vi "Drivetrain Loop.vi"(6 "Reset the clock":bool, 8 "In 4":dbl, 9 "In 3":dbl, 10 "In 2":dbl, 11 "In 1":dbl) -> (0 "Out 4":dbl, 1 "Out 3":dbl, 2 "Out 2":dbl, 3 "Out 1":dbl)   [LabVIEW 2015]
uses:
  Common Code/Drivetrain Modes.ctl
  Common Code/Change Detect Boolean.vi
  Robot Global Data.vi
  <vilib>/Rock Robotics/WPI/Solenoid/Deprecated/WPI_SolenoidSetBool.vi
panel:
  out "Modes":T1=enum."Goal Vision Targeting"
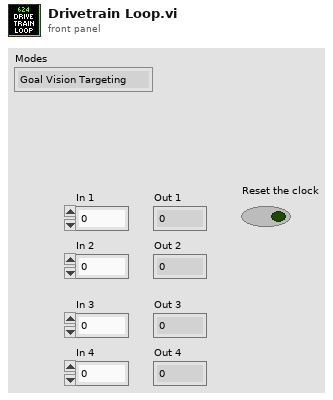
[diagram p1: front panel]
types:
  T1 = typedef "Drivetrain Modes.ctl" = enum16{"Tank", "Climb", "Manual", "Goal Vision Targeting", "PID Distance Drive", "Hybrid", "Gyro Steer"}
  T2 = typedef "Drivetrain Commands.ctl" = cluster{"Y Power":dbl, "Turn Power":dbl, "2nd Gear?":bool, "Modes":T1, "Heading Target":dbl, "X Max Speed":dbl, "Y Max Speed":dbl, "X Min Speed":dbl, "Y Min Speed":dbl, "Y Target":dbl, "Max Accel":dbl, "Max Velocity":dbl, "Y Power 2":dbl, "Pivot Speed":dbl}
  T3 = typedef "WPI_DriverStationRobotMode2.ctl" = enum16{"Autonomous Disabled", "Autonomous Enabled", "Teleop Disabled", "Teleop Enabled", "Disconnected", "Finish", "Test Disabled", "Test Enabled", "Emergency Stopped"}
  T4 = typedef "Goal Vision Packet.ctl" = cluster{"Distance":dbl, "Center X":dbl, "Center Y":dbl, "Found Target?":bool, "Robot Center":dbl, "Angle":dbl}
  T5 = typedef "Dashboard Control Data.ctl" = cluster{"Shooter Presets":T6, "Encoder Control":T8, "Steer PID output":cluster{"output high":dbl, "output low":dbl}, " Steer PID gains":cluster{"proportional gain (Kc)":dbl, "integral time (Ti, min)":dbl, "derivative time (Td, min)":dbl}, "Drivetrain Settings":T9, "Vision Packet":T4, "Dashboard Drivetrain Command":T10, "Info/Command Cluster":T12, "Ball Vision Packet":T13, "Intake Presets":T15, "Intake Encoder Control":T17, "Climb Presets":T18, "Goal Output Range":cluster{"output high":dbl, "output low":dbl}, "Enabled Systems":T19, "Auton Presets":T20, "Pressure M":dbl, "Pressure B":dbl, "Vision Timeout":dbl, "Auto-Shift":T21}
  T6 = typedef "Shooter Presets.ctl" = cluster{"Batter Shot":T7, "Deep Middle":T7, "Manual Shot":T7, "Left Ticks Per Rotation":dbl, "Right Ticks Per Rotation":dbl, "Low Bar Shot":T7, "Shooter RPM Tolerance":dbl, "Trigger Power":dbl, "Fire from Load Delay":i32, "Max Angle":dbl, "Min Angle":dbl, "Angle PID gains":cluster{"P":dbl, "I":dbl, "D":dbl}, "Angle Output":cluster{"output high":dbl, "output low":dbl}, "Shooter Angle Tolerance":dbl, "Vision Shoot x^2":dbl, "Vision Shoot x":dbl, "Feed Forward Max Accel":dbl, "Feed Forward Kv":dbl, "Backwards Trigger":dbl, "Shot Finish Delay (ms)":dbl, "Angle Max Current":dbl, "Angle Current Trip Time":dbl, "Intake Angle":dbl, "Vision Shoot c":dbl, "Reset?":bool, "Button Release Delay":dbl, "Angle Pot x":dbl, "Angle Pot c":dbl, "Ignore Angle?":bool, "Max RPM":dbl, "Safty Frist Angle":dbl, "Intake Danger Height":dbl, "Angle Pot B":i32, "Angle Pot M":dbl, "FF Finish RPM":dbl, "RPM PID Right":cluster{"P":dbl, "I":dbl, "D":dbl, "FF":dbl}, "RPM PID Left":cluster{"P":dbl, "I":dbl, "D":dbl, "FF":dbl}, "Backwards RPM":dbl, "Vision RPM":dbl, "Run Wheels Backward Delay":u32, "Cleat Shot":T7, "Vision Far RPM":dbl, "Vision Far Distance":dbl, "Vision Far Angle":dbl}
  T7 = typedef "Shot Presets.ctl" = cluster{"L":dbl, "R":dbl, "A":dbl}
  T8 = typedef "Encoder Control.ctl" = cluster{"Right Tick Constant":dbl, "Left Tick Constant":dbl, "Reset?":bool, "Y Dist":cluster{"PID gains":cluster{"proportional gain (Kc)":dbl, "integral time (Ti, min)":dbl, "derivative time (Td, min)":dbl}}, "Y Stop Thresh":dbl, "Y Stop Speed":dbl}
  T9 = typedef "Drivetrain Settings.ctl" = cluster{"Gyro Tolerance":dbl, "Throttle Ramp (ms)":dbl, "Kv":dbl, "Ka":dbl, "Feed Forward P":dbl, "Feed Forward D":dbl, "Goal Vision PID gains":cluster{"proportional gain (Kc)":dbl, "integral time (Ti, min)":dbl, "derivative time (Td, min)":dbl}, "Goal Detection Window":dbl, "Creep Rate":dbl, "Vision Throttle Threshold":dbl, "Min Turn Output":dbl, "Left Batter Angle":dbl, "Right Batter Angle":dbl}
  T10 = typedef "Dashboard Drivetrain Command.ctl" = cluster{"Drivetrain Vision":T11}
  T11 = typedef "Drivetrain Vision.ctl" = cluster{"Goal Window":dbl, "Ball Window":dbl}
  T12 = typedef "Ball Tracking Command Cluster.ctl" = cluster{"Distance to Ball":dbl, "Desired Angle":dbl, "Command":enum16{"Turn to Ball", "Turn to Angle", "Get Distance"}, "Pixels from Center":dbl}
  T13 = typedef "Ball Vision Packet.ctl" = cluster{"Ball Detected?":bool, "Distance to Ball":dbl, "Desired Angle":dbl, "Pixels from Center":dbl, "Tracking mode":T14}
  T14 = typedef "Tracking Mode.ctl" = enum16{"Turn to Ball", "Turn to Angle"}
  T15 = typedef "Intake Presets.ctl" = cluster{"Intake Speed":dbl, "Outake Speed":dbl, "Low Height":dbl, "Half Height":dbl, "High Idle Height":dbl, "Angle Speed":dbl, "Angle Tolerance":dbl, "Encoder Scale":dbl, "Load Height":dbl, "Output Range":T16, "Rotation Power Max/Min":dbl, "MaxCurrent":dbl, "Intake Trip Time":dbl, "Idle Height":dbl, "Max Height":dbl, "Reset Encoders?":bool, "PID gains":cluster{"proportional gain (Kc)":dbl, "integral time (Ti, min)":dbl, "derivative time (Td, min)":dbl}, "Intake Stop Delay":u32, "Settle Time":dbl, "Settle Wait Time":dbl, "Pull Up Delay":dbl}
  T16 = typedef "Drivetrain Output Range.ctl" = cluster{"output high":dbl, "output low":dbl}
  T17 = typedef "IntakeEcoderControl.ctl" = cluster{"Arm Tick Constant":dbl, "Reset?":bool, "Y Dist":cluster{"PID gains":cluster{"proportional gain (Kc)":dbl, "integral time (Ti, min)":dbl, "derivative time (Td, min)":dbl}}, "Y Stop Thresh":dbl, "Y Stop Speed":dbl}
  T18 = typedef "Climb Presets.ctl" = cluster{"Pull Power":dbl, "Extend Power":dbl}
  T19 = typedef "Enabled Systems.ctl" = cluster{"Shoot":bool, "Intake":bool, "DT":bool, "Gyro":bool, "100ms":bool, "US":bool}
  T20 = typedef "Autonomous Presets.ctl" = cluster{"Pitch Limit":dbl, "Roll Limit":dbl, "Start Position":dbl, "Cross Position":dbl}
  T21 = typedef "Auto Shift Cluster.ctl" = cluster{"Delay":dbl, "Speed Thresh":dbl, "Upshift Accel":dbl, "Upshift Throttle":dbl, "Upshift Throttle Accel":dbl, "Downshift Throttle":dbl, "Downshift Throttle Accel":dbl, "Pressure Threshold":dbl}
  T22 = typedef "Dist Drive Status.ctl" = cluster{"Y In Range":bool, "X In Range":bool, "Gyro In Range":bool, "Y Dist":dbl, "X Dist":dbl, "Gyro":dbl}
  T23 = typedef "WPI_MotorControlDeviceRef.ctl" = cluster{"DeviceStatus":errorcluster, "Type":T24, "PWM":cluster{"PWM Channel":T25, "DeadBand":T26}, "CAN":cluster{"Device Number":u8, "Control Mode":T27, "Semaphore":T28, "Max Vout":dbl, "TalonSRX Control Mode":T29}, "Invert":bool}
  T24 = typedef "WPI_MotorControlType.ctl" = enum16{"PWM", "CAN", "CANTalonSRX"}
  T25 = typedef "FPGA_DIOPWMChannel.ctl" = enum8{"PWM 0", "PWM 1", "PWM 2", "PWM 3", "PWM 4", "PWM 5", "PWM 6", "PWM 7", "PWM 8", "PWM 9", "PWM MXP 0", "PWM MXP 1", "PWM MXP 2", "PWM MXP 3", "PWM MXP 4", "PWM MXP 5", "PWM MXP 6", "PWM MXP 7", "PWM MXP 8", "PWM MXP 9", "Invalid"}
  T26 = typedef "WPI_PWMDeadband.ctl" = cluster{"Name":string, "maxPositivePwm":i32, "minPositivePwm":i32, "centerPwm":i32, "maxNegativePwm":i32, "minNegativePwm":i32, "angularRange":u16}
  T27 = typedef "WPI_CANJaguar_ControlMode.ctl" = enum8{"Percent VBus", "Current", "Speed", "Position", "Voltage"}
  T28 = typedef "Semaphore RefNum" = refnum<k1>
  T29 = typedef "WPI_CANTalonSRX_APIControlMode.ctl" = enum8{"Percent VBus", "Speed", "Position", "Slave", "Unchanged / Invalid", "Voltage Compensation", "Current", "Motion Profile"}
  T30 = typedef "WPI_SolenoidDevRef.ctl" = cluster{"DevStatus":errorcluster, "Pneumatics Control Module":u8, "Forward Solenoid Channel":T31, "Reverse Solenoid Channel":T31}
  T31 = typedef "WPI_SolenoidChannel.ctl" = enum8{"Solenoid 0", "Solenoid 1", "Solenoid 2", "Solenoid 3", "Solenoid 4", "Solenoid 5", "Solenoid 6", "Solenoid 7", "Invalid"}
  T32 = typedef "Drivetrain Status Cluster.ctl" = cluster{"Modes":T1, "Y (Throttle)":dbl, "X (Steer)":dbl, "Gyro In Range?":bool, "Distance Drive Finished?":bool, "Stop Eject Lockout":bool, "Dist Drive Status":T22, "Y Target":dbl, "Heading Target":dbl, "Vision Target Aligned?":bool, "Gear":dbl, "1st Gear Time":dbl, "2nd Gear Time":dbl, "1st Gear Shifts":dbl, "2nd Gear Shifts":dbl}
  T33 = typedef "Climb Status Cluster.ctl" = cluster{"Pull Power":dbl, "Unpin Power":dbl, "PTO Engaged?":bool, "Climb Mode":T34}
  T34 = typedef "Climb Mode.ctl" = enum16{"Auto", "Semi-Auto", "Manual"}
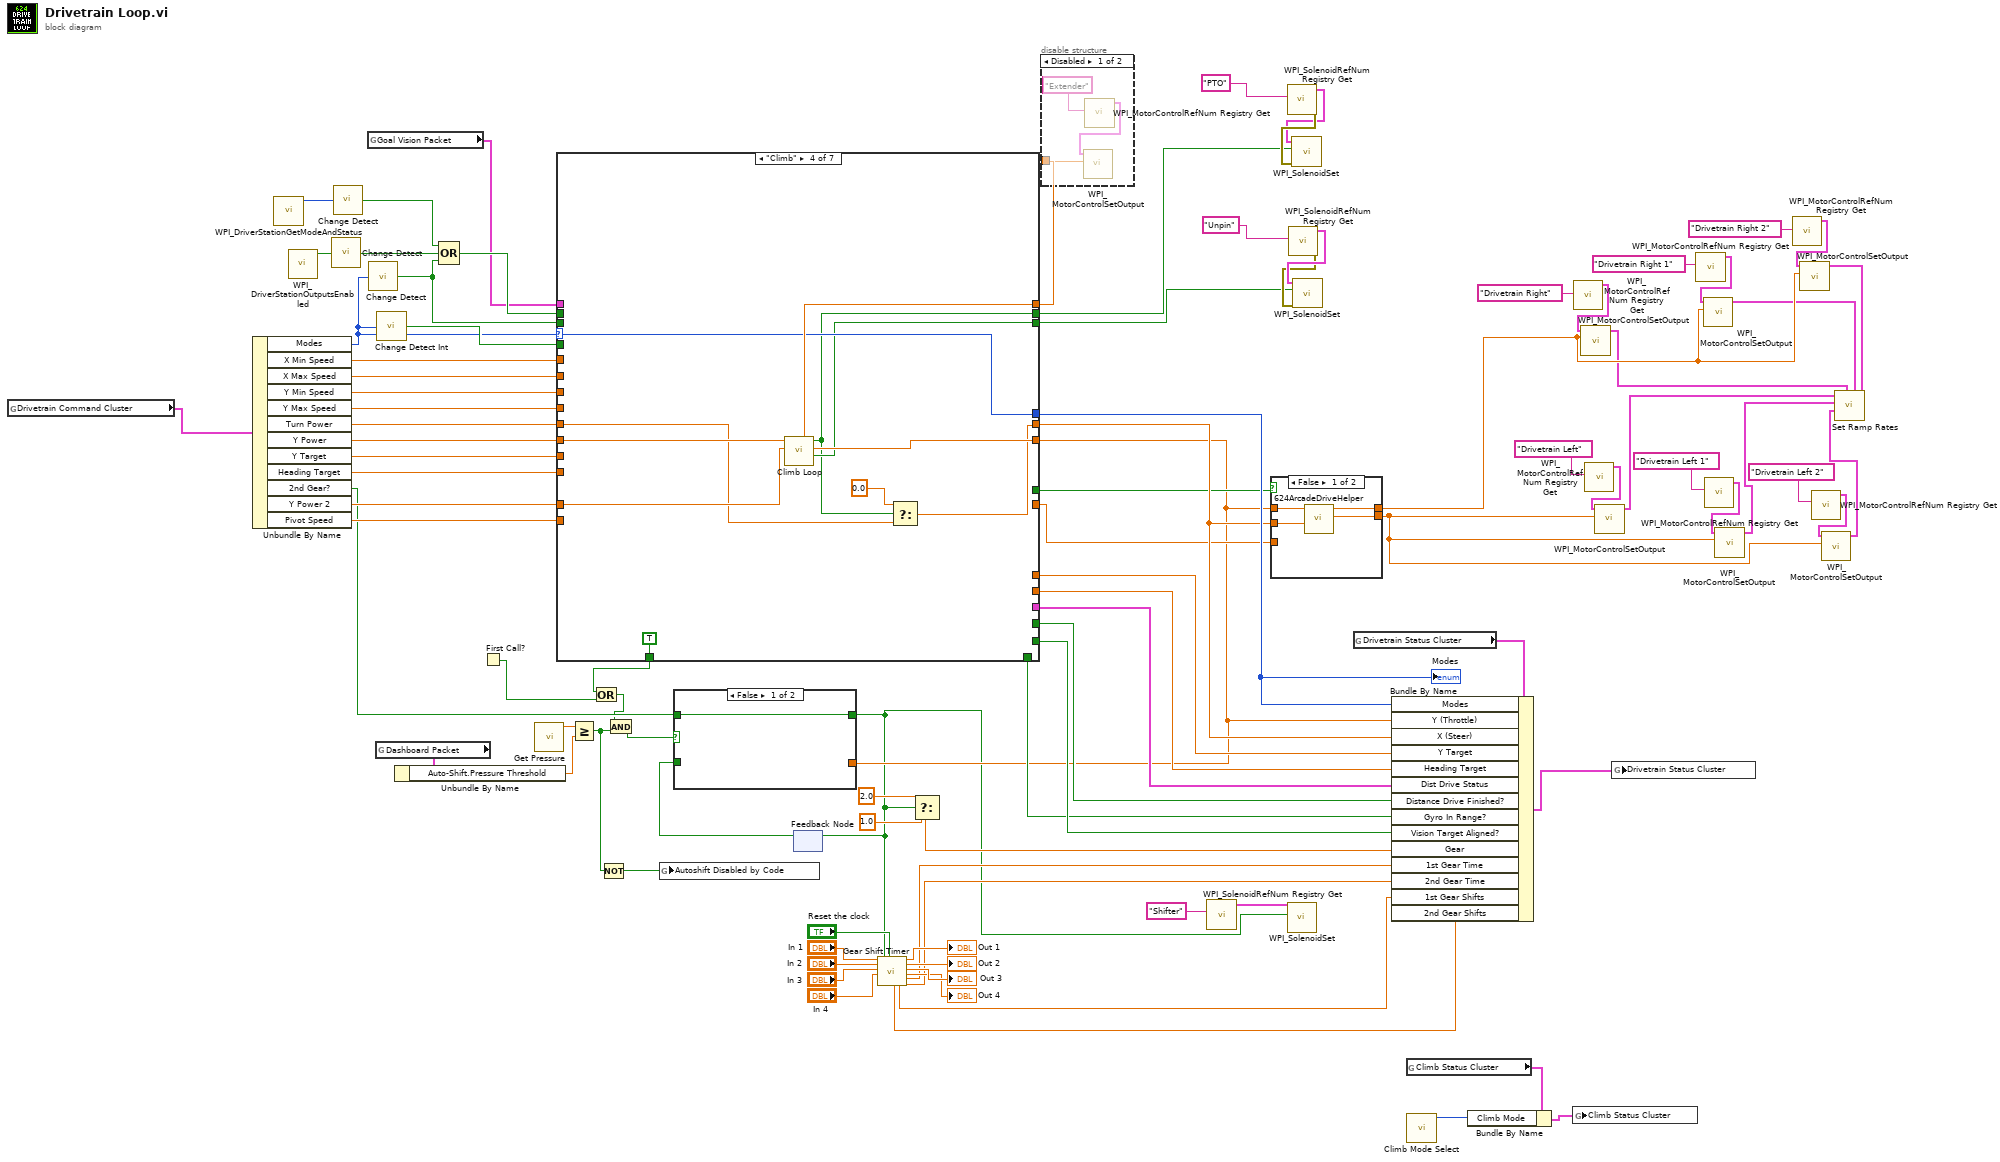
[diagram p0: block diagram]
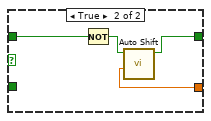
[diagram p2: hidden frame]
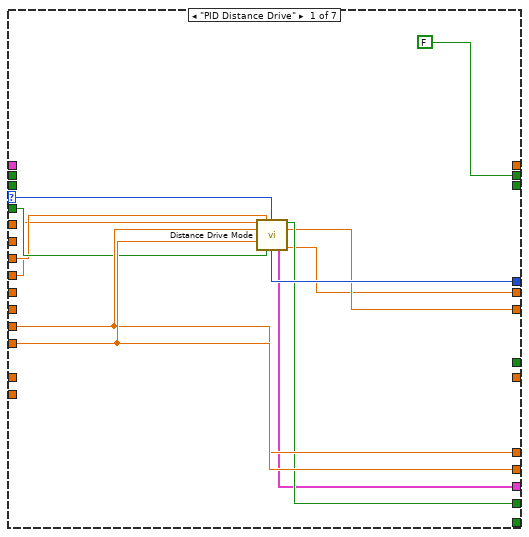
[diagram p4: hidden frame]
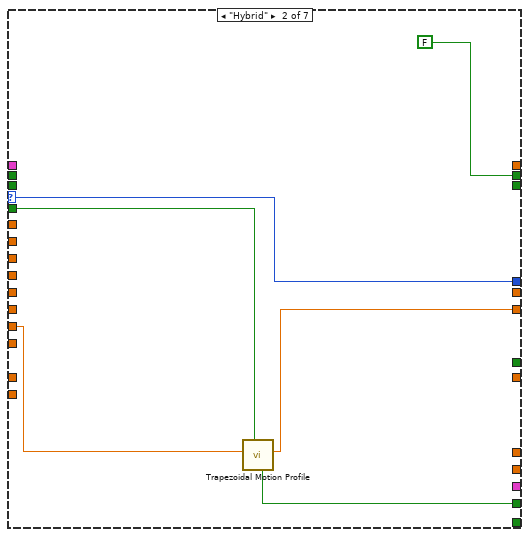
[diagram p5: hidden frame]
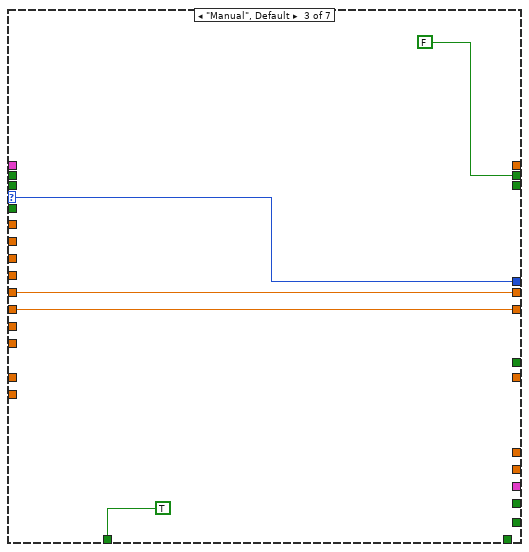
[diagram p6: hidden frame]
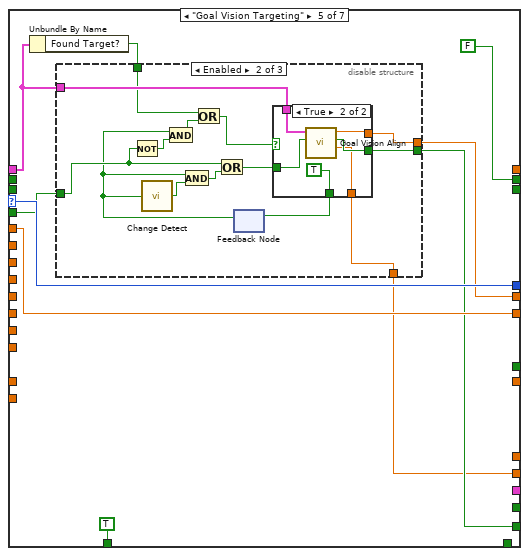
[diagram p7: hidden frame]
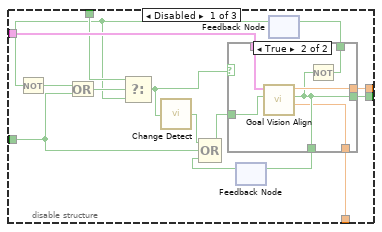
[diagram p8: hidden frame]
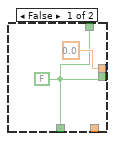
[diagram p9: hidden frame]
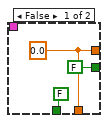
[diagram p10: hidden frame]
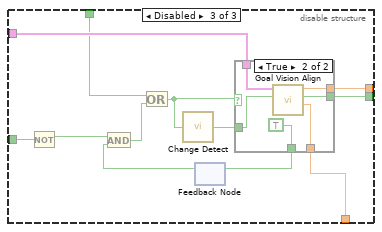
[diagram p11: hidden frame]
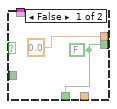
[diagram p12: hidden frame]
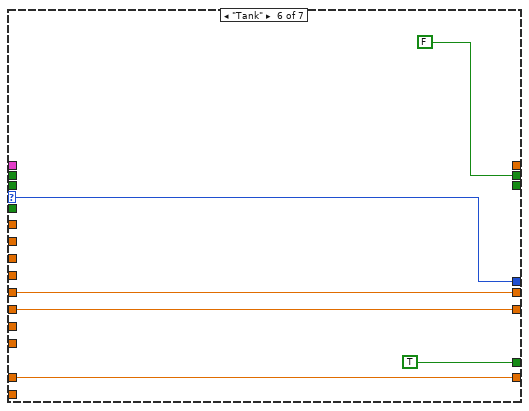
[diagram p13: hidden frame]
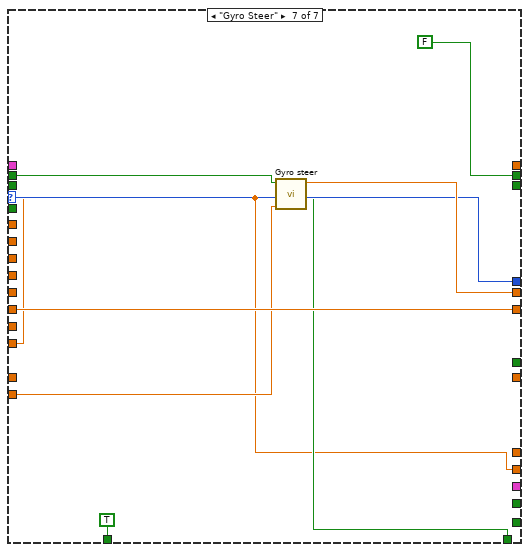
[diagram p14: hidden frame]
diagram:
  n1 = global read "Robot Global Data.vi" "Drivetrain Command Cluster"() -> (w60:T2)
  n2 = Unbundle By Name(w60) -> ("Modes"=w45:T1, "X Min Speed"=w69:dbl, "X Max Speed"=w68:dbl, "Y Min Speed"=w67:dbl, "Y Max Speed"=w66:dbl, "Turn Power"=w65:dbl, "Y Power"=w64:dbl, "Y Target"=w63:dbl, "Heading Target"=w62:dbl, "2nd Gear?"=w13:bool, "Y Power 2"=w61:dbl, "Pivot Speed"=w46:dbl)
  n3 = call <vilib>:"WPI_DriverStationGetModeAndStatus.vi"() -> ("Robot Mode"=w28:T3)  [unwired: 10 in, 1 out]
  n4 = call <vilib>:"WPI_DriverStationOutputsEnabled.vi"() -> ("OutputsEnabled?"=w30:bool)  [unwired: 10 in, 1 out]
  n5 = call-poly "Change Detect.vi"("In"=w30) -> ("Changed?"=w29:bool)
  n6 = call-poly "Change Detect.vi"("In"=w28) -> ("Changed?"=w27:bool)
  n7 = global read "Robot Global Data.vi" "Goal Vision Packet"() -> (w14:T4)
  n8 = call-poly "Change Detect.vi"("In"=w45) -> ("Changed?"=w26:bool)
  n9 = global read "Robot Global Data.vi" "Dashboard Packet"() -> (w8:T5)
  n10 = call "Change Detect Int.vi"("In"=w45) -> ("Changed?"=w90:bool)
  n11 = Unbundle By Name(w8) -> ("Auto-Shift.Pressure Threshold"=w7:dbl)
  n12 = Compound Arithmetic op=OR(w27, w29, w26) -> (w44:bool)
  n13 = First Call?() -> (First Call?: T/F=w3:bool)
  n14 = call "Get Pressure.vi"() -> ("Pressure"=w9:dbl)  [unwired: 10 in, 1 out]
  n15 = case shown="\"Climb\"" w45 {
    selector: w45 -> [w106 w107 w117 w126 w138 w206 w214]
    tunnel: w69 -> [_ _ _ _ w136 _ _]
    tunnel: w68 -> [_ _ _ _ _ _ _]
    tunnel: w67 -> [w97 _ _ _ _ _ _]
    tunnel: [w101 w112 w116 w128 w136 w210 w217] -> w12
    tunnel: [w99 _ w114 w121 w135 w208 w218] -> w43
    tunnel: [w106 w107 w117 w126 w138 w206 w214] -> w93
    tunnel: w90 -> [w98 w110 _ _ w130 _ _]
    tunnel: [_ _ _ _ w134 _ _] -> w84
    tunnel: [w100 _ _ _ _ _ _] -> w82
    tunnel: [w102 w111 _ _ _ _ _] -> w83
    tunnel: [w104 _ _ _ _ _ _] -> w81
    tunnel: [w105 _ _ _ w131 _ w212] -> w80
    tunnel: w66 -> [w96 _ _ _ _ _ _]
    tunnel: w65 -> [_ _ w114 w119 _ w208 _]
    tunnel: w64 -> [_ _ w116 w125 _ w210 w217]
    tunnel: w62 -> [w105 _ _ _ _ _ w212]
    tunnel: w63 -> [w104 w109 _ _ _ _ _]
    tunnel: w14 -> [_ _ _ _ w133 _ _]
    tunnel: [_ _ _ w127 _ _ _] -> w70
    tunnel: [FALSE ("PTO Engage") FALSE ("PTO Engage") FALSE ("PTO Engage") w122 FALSE ("PTO Engage") FALSE ("PTO Engage") FALSE ("PTO Engage")] -> w74
    tunnel: w61 -> [_ _ _ w124 _ w209 _]
    tunnel: [_ _ _ _ _ w209 _] -> w31
    tunnel: w46 -> [_ _ _ _ _ _ w216]
    tunnel: w44 -> [_ _ _ _ _ _ w215]
    tunnel: [_ _ _ _ _ TRUE _] -> w32
    tunnel: w26 -> [_ _ _ _ _ _ _]
    tunnel: [_ _ _ _ _ _ w213] -> w25
    tunnel: [_ _ _ w123 _ _ _] -> w21
    tunnel: [_ _ TRUE TRUE TRUE _ TRUE] -> w4
    frame "PID Distance Drive" {
      n16 = call "Distance Drive Mode.vi"("Y Output High"=w96, "Y Output Low"=w97, "Y target"=w104, "Heading target"=w105, "Reinitialize"=w98) -> ("isFinished"=w102:bool, "Y out"=w101:dbl, "Dist Drive Status"=w100:T22, "X out"=w99:dbl)  [unwired: 7 in]
    }
    frame "Hybrid" {
      n17 = call "Trapezoidal Motion Profile.vi"("Reset?"=w110, "Distance"=w109) -> ("Throttle Out"=w112:sgl, "Finished?"=w111:bool)  [unwired: 8 in]
    }
    frame "Manual", Default {
    }
    frame "Climb" {
      n18 = call "Climb Loop.vi"("Extend Power in"=w124, "Y Power"=w125) -> ("Unpin?"=w123:bool, "Pull Power"=w128:dbl, "PTO Engaged?"=w122:bool, "Extend Power"=w127:dbl)  [unwired: 6 in]
      n19 = Select(t=0.0, s=w122, f=w119) -> (s? t:f=w121:dbl)
    }
    frame "Goal Vision Targeting" {
      n20 = Unbundle By Name(w133) -> ("Found Target?"=w132:bool)
      n21 = disable-structure shown="Enabled" {
        disable-tunnel: [w153 w172 w195] -> w135
        disable-tunnel: [w152 w168 w196] -> w134
        disable-tunnel: w133 -> [w151 w175 w193]
        disable-tunnel: w132 -> [w148 w174 w187]
        disable-tunnel: [w142 w167 w194] -> w131
        disable-tunnel: w130 -> [w141 w166 w191]
        frame Disabled {
          n22 = feedback #1() -> (w139:bool)  [unwired: 1 in]
          n23 = feedback #2() -> (w147:bool)  [unwired: 1 in]
          n24 = Not(x=w147) -> (.not. x?=w150:bool)
          n25 = Or(x=w150, y=w141) -> (x .or. y?=w149:bool)
          n26 = Select(t=w148, s=w149, f=w147) -> (s? t:f=w146:bool)
          n27 = call-poly "Change Detect.vi"("In"=w146) -> ("Changed?"=w144:bool)
          n28 = Compound Arithmetic op=OR(w144, w141, w139) -> (w143:bool)
          n29 = case shown="True" w146 {
            tunnel: [0.0 ("Turn Power") w161] -> w153
            tunnel: [w154 w157] -> w152
            tunnel: w151 -> [_ w160]
            tunnel: w143 -> [_ w159]
            tunnel: [w154 w158] -> w145
            tunnel: [w154 w157] -> w140
            tunnel: [_ w156] -> w142
            frame False {
              w154 = FALSE ("Aligned?")
            }
            frame True {
              n30 = call "Goal Vision Align.vi"("reinitialize? (F)"=w159, "Goal Vision Packet"=w160) -> ("Heading Target"=w156:dbl, "Aligned?"=w157:bool, "Turn Power"=w161:dbl)  [unwired: 7 in]
              n31 = Not(x=w157) -> (.not. x?=w158:bool)
            }
          }
          n32 = feedback-in #1(w140) -> ()
          n33 = feedback-in #2(w145) -> ()
        }
        frame Enabled {
          n34 = Not(x=w166) -> (.not. x?=w164:bool)
          n35 = feedback #3() -> (w163:bool)  [unwired: 1 in]
          n36 = call-poly "Change Detect.vi"("In"=w163) -> ("Changed?"=w171:bool)
          n37 = And(x=w163, y=w164) -> (x .and. y?=w162:bool)
          n38 = And(x=w163, y=w171) -> (x .and. y?=w170:bool)
          n39 = Or(x=w174, y=w162) -> (x .or. y?=w165:bool)
          n40 = Or(x=w166, y=w170) -> (x .or. y?=w169:bool)
          n41 = case shown="True" w165 {
            tunnel: [w177 w181] -> w172
            tunnel: [FALSE ("Aligned?") TRUE] -> w173
            tunnel: w175 -> [_ w183]
            tunnel: w169 -> [_ w182]
            tunnel: [FALSE ("Aligned?") w180] -> w168
            tunnel: [w177 w179] -> w167
            frame False {
              w177 = 0.0 ("Turn Power")
            }
            frame True {
              n42 = call "Goal Vision Align.vi"("reinitialize? (F)"=w182, "Goal Vision Packet"=w183) -> ("Heading Target"=w179:dbl, "Aligned?"=w180:bool, "Turn Power"=w181:dbl)  [unwired: 7 in]
            }
          }
          n43 = feedback-in #3(w173) -> ()
        }
        frame Disabled {
          n44 = Not(x=w191) -> (.not. x?=w190:bool)
          n45 = feedback #4() -> (w189:bool)  [unwired: 1 in]
          n46 = And(x=w190, y=w189) -> (x .and. y?=w188:bool)
          n47 = Or(x=w187, y=w188) -> (x .or. y?=w186:bool)
          n48 = call-poly "Change Detect.vi"("In"=w186) -> ("Changed?"=w185:bool)
          n49 = case shown="True" w186 {
            tunnel: [w197 w204] -> w196
            tunnel: [0.0 ("Turn Power") w203] -> w195
            tunnel: [_ w202] -> w194
            tunnel: w193 -> [_ w201]
            tunnel: [w197 TRUE] -> w192
            tunnel: w185 -> [_ w199]
            frame False {
              w197 = FALSE ("Aligned?")
            }
            frame True {
              n50 = call "Goal Vision Align.vi"("reinitialize? (F)"=w199, "Goal Vision Packet"=w201) -> ("Heading Target"=w202:dbl, "Aligned?"=w204:bool, "Turn Power"=w203:dbl)  [unwired: 7 in]
            }
          }
          n51 = feedback-in #4(w192) -> ()
        }
      }
    }
    frame "Tank" {
    }
    frame "Gyro Steer" {
      n52 = call "Gyro steer.vi"("Turn Speed"=w216, "Target Angle"=w212, "Changed?"=w215) -> ("In Range?"=w213:bool, "X out"=w218:dbl)  [unwired: 7 in]
    }
  }
  "Modes" <- w93
  n53 = Greater Or Equal?(x=w9, y=w7) -> (x >= y?=w1:bool)
  n54 = Or(x=w4, y=w3) -> (x .or. y?=w2:bool)
  n55 = Not(x=w1) -> (.not. x?=w6:bool)
  n56 = And(x=w2, y=w1) -> (x .and. y?=w5:bool)
  n57 = global write "Robot Global Data.vi" "Autoshift Disabled by Code"(w6) -> ()
  n58 = feedback #5() -> (w10:bool)  [unwired: 1 in]
  n59 = case shown="False" w5 {
    tunnel: w13 -> [w220 w224]
    tunnel: [w220 w223] -> w11
    tunnel: w12 -> [_ w222]
    tunnel: w10 -> [_ _]
    frame False {
    }
    frame True {
      n60 = Not(x=w224) -> (.not. x?=w221:bool)
      n61 = call "Auto Shift.vi"("Throttle"=w222, "Manual Low Gear"=w221) -> ("High Gear"=w223:bool)  [unwired: 9 in]
    }
  }
  n62 = feedback-in #5(w11) -> ()
  n63 = call "Gear Shift Timer.vi"("In 1"="In 1", "In 2"="In 2", "In 3"="In 3", "In 4"="In 4", "1st Gear?"=w11, "RESET THE CLOCKS"="Reset the clock") -> ("2nd Gear Shifts"=w59:dbl, "1st Gear Shifts"=w58:dbl, "Out 1"=→"Out 1":dbl, "Out 2"=→"Out 2":dbl, "Out 3"=→"Out 3":dbl, "Out 4"=→"Out 4":dbl, "1st Gear Time"=w53:dbl, "2nd Gear Time"=w52:dbl)  [unwired: 6 in]
  n64 = Select(t=2.0, s=w11, f=1.0) -> (s? t:f=w79:dbl)
  n65 = disable-structure shown="Disabled" {
    disable-tunnel: w70 -> [w227 _]
    frame Disabled {
      n66 = call <vilib>:"WPI_MotorControlRefNum Registry Get.vi"("refnum name"="Extender") -> ("MotorControlDevRef"=w226:T23)  [unwired: 9 in, 1 out]
      n67 = call <vilib>:"WPI_MotorControlSetOutput.vi"("Output"=w227, "MotorControlDevRef"=w226) -> ()  [unwired: 7 in, 3 out]
    }
    frame Enabled {
    }
  }
  n68 = call <vilib>:"WPI_SolenoidRefNum Registry Get.vi"("refnum name"="Shifter") -> ("SolenoidDevRef"=w94:T30)  [unwired: 9 in, 1 out]
  n69 = case shown="False" w32 {
    tunnel: w43 -> [w231 _]
    tunnel: w12 -> [w230 w233]
    tunnel: [w229 w233] -> w38
    tunnel: [w228 w232] -> w33
    tunnel: w31 -> [_ w232]
    frame False {
      n70 = call "624ArcadeDriveHelper.vi"("Turn Power"=w231, "Y Power"=w230) -> ("Left"=w229:dbl, "Right"=w228:dbl)  [unwired: 8 in]
    }
    frame True {
    }
  }
  n71 = call <vilib>:"WPI_SolenoidRefNum Registry Get.vi"("refnum name"="PTO") -> ("error out"=w77:errorcluster, "SolenoidDevRef"=w76:T30)  [unwired: 9 in]
  n72 = call-poly <vilib>:"WPI_SolenoidSet.vi"("Value"=w11, "SolenoidDevRef"=w94) -> ()  [unwired: 8 in, 2 out]
  n73 = call <vilib>:"WPI_SolenoidRefNum Registry Get.vi"("refnum name"="Unpin") -> ("error out"=w22:errorcluster, "SolenoidDevRef"=w23:T30)  [unwired: 9 in]
  n74 = call-poly <vilib>:"WPI_SolenoidSet.vi"("error in (no error)"=w77, "Value"=w74, "SolenoidDevRef"=w76) -> ()  [unwired: 7 in, 2 out]
  n75 = call-poly <vilib>:"WPI_SolenoidSet.vi"("error in (no error)"=w22, "Value"=w21, "SolenoidDevRef"=w23) -> ()  [unwired: 7 in, 2 out]
  n76 = global read "Robot Global Data.vi" "Drivetrain Status Cluster"() -> (w78:T32)
  n77 = Bundle By Name(cluster=w78, "Modes"=w93, "Y (Throttle)"=w12, "X (Steer)"=w43, "Y Target"=w81, "Heading Target"=w80, "Dist Drive Status"=w82, "Distance Drive Finished?"=w83, "Gyro In Range?"=w25, "Vision Target Aligned?"=w84, "Gear"=w79, "1st Gear Time"=w53, "2nd Gear Time"=w52, "1st Gear Shifts"=w58, "2nd Gear Shifts"=w59) -> (w85:T32)
  n78 = global read "Robot Global Data.vi" "Climb Status Cluster"() -> (w71:T33)
  n79 = call "Climb Mode Select.vi"() -> ("Mode"=w72:T34)  [unwired: 11 in]
  n80 = Bundle By Name(cluster=w71, "Climb Mode"=w72) -> (w73:T33)
  n81 = global write "Robot Global Data.vi" "Climb Status Cluster"(w73) -> ()
  n82 = call <vilib>:"WPI_MotorControlRefNum Registry Get.vi"("refnum name"="Drivetrain Right") -> ("MotorControlDevRef"=w89:T23)  [unwired: 9 in, 1 out]
  n83 = call <vilib>:"WPI_MotorControlSetOutput.vi"("Output"=w33, "MotorControlDevRef"=w89) -> ("MotorControlDevRef"=w17:T23)  [unwired: 7 in, 2 out]
  n84 = call <vilib>:"WPI_MotorControlRefNum Registry Get.vi"("refnum name"="Drivetrain Left") -> ("MotorControlDevRef"=w88:T23)  [unwired: 9 in, 1 out]
  n85 = call <vilib>:"WPI_MotorControlSetOutput.vi"("Output"=w38, "MotorControlDevRef"=w88) -> ("MotorControlDevRef"=w20:T23)  [unwired: 7 in, 2 out]
  n86 = global write "Robot Global Data.vi" "Drivetrain Status Cluster"(w85) -> ()
  n87 = call <vilib>:"WPI_MotorControlRefNum Registry Get.vi"("refnum name"="Drivetrain Right 1") -> ("MotorControlDevRef"=w37:T23)  [unwired: 9 in, 1 out]
  n88 = call <vilib>:"WPI_MotorControlSetOutput.vi"("Output"=w33, "MotorControlDevRef"=w37) -> ("MotorControlDevRef"=w16:T23)  [unwired: 7 in, 2 out]
  n89 = call <vilib>:"WPI_MotorControlRefNum Registry Get.vi"("refnum name"="Drivetrain Left 1") -> ("MotorControlDevRef"=w42:T23)  [unwired: 9 in, 1 out]
  n90 = call <vilib>:"WPI_MotorControlSetOutput.vi"("Output"=w38, "MotorControlDevRef"=w42) -> ("MotorControlDevRef"=w19:T23)  [unwired: 7 in, 2 out]
  n91 = call <vilib>:"WPI_MotorControlRefNum Registry Get.vi"("refnum name"="Drivetrain Right 2") -> ("MotorControlDevRef"=w34:T23)  [unwired: 9 in, 1 out]
  n92 = call <vilib>:"WPI_MotorControlSetOutput.vi"("Output"=w33, "MotorControlDevRef"=w34) -> ("MotorControlDevRef"=w15:T23)  [unwired: 7 in, 2 out]
  n93 = call <vilib>:"WPI_MotorControlRefNum Registry Get.vi"("refnum name"="Drivetrain Left 2") -> ("MotorControlDevRef"=w39:T23)  [unwired: 9 in, 1 out]
  n94 = call <vilib>:"WPI_MotorControlSetOutput.vi"("Output"=w38, "MotorControlDevRef"=w39) -> ("MotorControlDevRef"=w18:T23)  [unwired: 7 in, 2 out]
  n95 = call "Set Ramp Rates.vi"("DT Right 2"=w15, "DT Right 1"=w16, "DT Right"=w17, "DT Left 2"=w18, "DT Left 1"=w19, "DT Left"=w20) -> ()  [unwired: 6 in]
